vi "Model - Set DB Record.vi"(8 "error in (no error)":errorcluster, 10 "DB Record":T1, 11 "View Model":T2) -> (0 "error out":errorcluster, 3 "View Model":T2)   [LabVIEW 2017]
doc: "Set actual DB Record value into DVR."
uses:
  Controls/View Model.ctl
  Controls/Shared Model.ctl
  Error/Controls/Error Model.ctl
  Error/Controls/Error Event.ctl
  Error/Controls/Error Type.ctl
  Configuration/Controls/Config DB Model.ctl
  Configuration/Controls/Config DB Command.ctl
  Configuration/Controls/Config DB Record.ctl
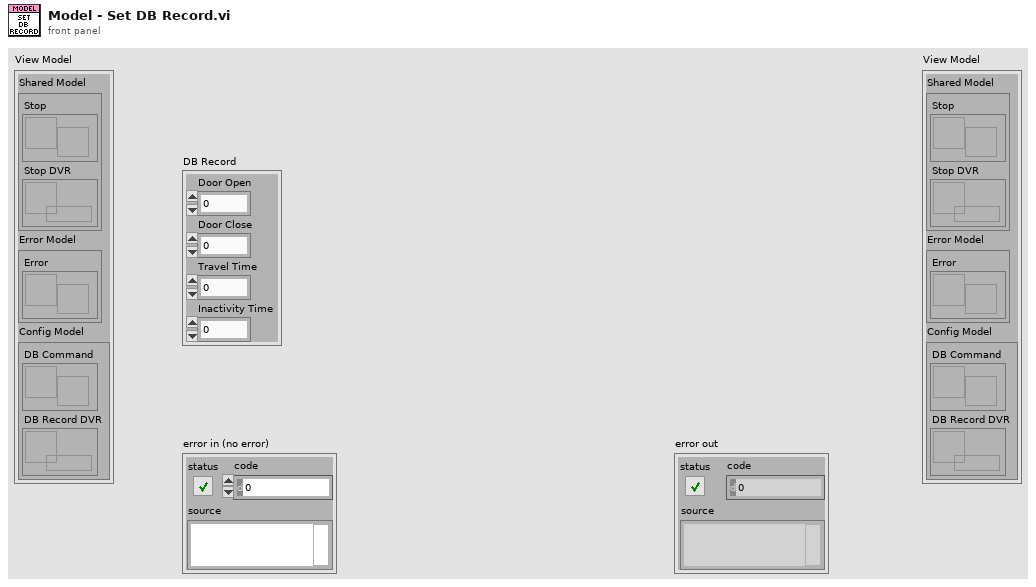
[diagram p1: front panel]
types:
  T1 = typedef "Config DB Record.ctl" = cluster{"Door Open":dbl, "Door Close":dbl, "Travel Time":dbl, "Inactivity Time":dbl}
  T2 = typedef "View Model.ctl" = cluster{"Shared Model":T3, "Error Model":T4, "Config Model":T5}
  T3 = typedef "Shared Model.ctl" = cluster{"Stop":refnum<user-event>, "Stop DVR":refnum<data-value>}
  T4 = typedef "Error Model.ctl" = cluster{"Error":refnum<user-event>}
  T5 = typedef "Config DB Model.ctl" = cluster{"DB Command":refnum<user-event>, "DB Record DVR":refnum<data-value>}
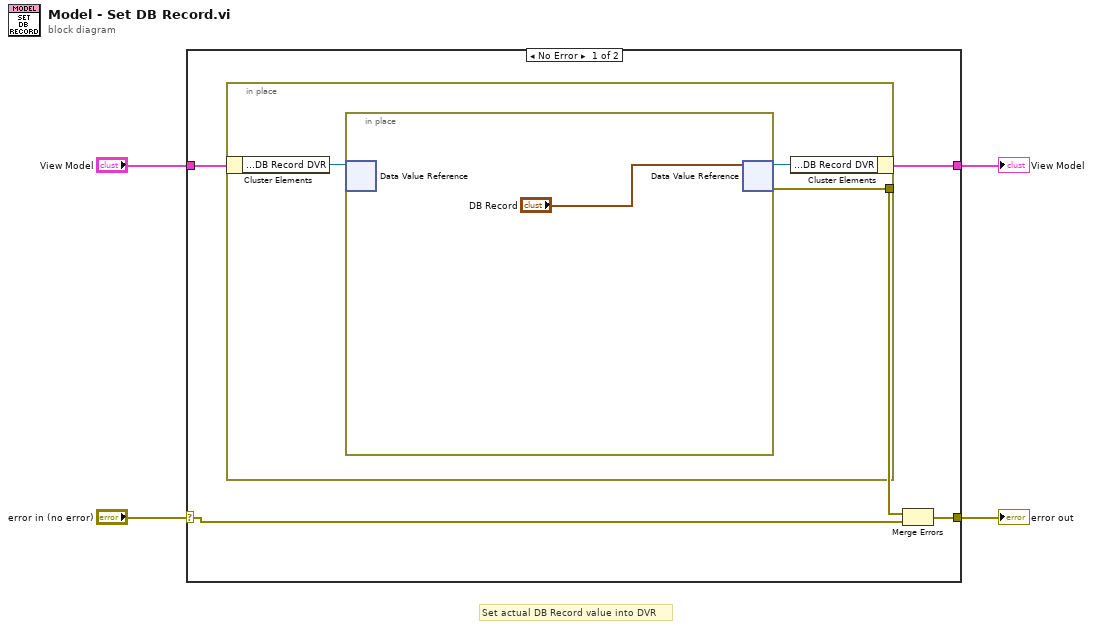
[diagram p0: block diagram]
diagram:
  # "Set actual DB Record value into DVR"
  n1 = case shown="No Error" "error in (no error)" {
    selector: "error in (no error)" -> [w7 w14]
    tunnel: "View Model" -> [w9 w15]
    tunnel: [w8 w15] -> w2
    tunnel: [w6 w14] -> w1
    frame No Error {
      n2 = in-place {
        in-place-border: [w10] -> w5
        n3 = in-place-cluster #1(w9) -> ("Config Model.DB Record DVR"=w12:refnum<data-value>)
        n4 = in-place {
          n5 = in-place-dvr #2(w12) -> ()  [unwired: 2 out]
          n6 = in-place-dvr #2("DB Record") -> (w11:refnum<data-value>, w10:errorcluster)
        }
        n7 = in-place-cluster #1("Config Model.DB Record DVR"=w11) -> (w8:T2)
      }
      n8 = Merge Errors(w5, w7) -> (w6:errorcluster)
    }
    frame Error {
    }
  }
  "error out" <- w1
  "View Model" <- w2
